vi "CRYGet Weight Name Array.vi"() -> (3 "Weighting Names":string[](array[string]))   [LabVIEW 2013]
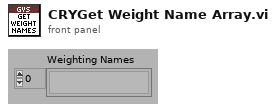
[diagram p1: front panel]
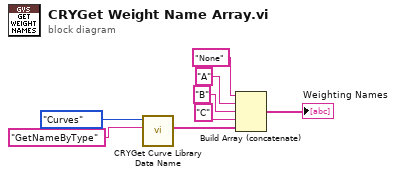
[diagram p0: block diagram]
diagram:
  n1 = call "CRYGet Curve Library Data Name.vi"("sAction"="GetNameByType", "Type"=enum16{"Curves", "Values", "Results", "WFM"}."Curves") -> ("sNames"=w6:string[])  [unwired: 6 in, 3 out]
  n2 = Build Array (concatenate)("None" ("String"), "A" ("String"), "B" ("String"), "C" ("String"), w6) -> (→"Weighting Names":string[])
